vi "Get Current Log File Info.vi"(8 "error in (no error)":errorcluster, 10 "Session Name in":string, 11 "Data Logging Manager Ref in":T1) -> (0 "error out":errorcluster, 1 "Log File Path":path, 2 "Session Name out":string, 3 "Data Logging Manager Ref out":T1, 4 "Start Time":timestamp, 5 "Size":i64)   [LabVIEW 2020, in "NI_VS Data Logging API.lvlib"]
doc: "Gets information about the file to which <B>Session Name in</B> is currently logging data. If the session is not actively logging data to a file, <B>Log File Path</B> returns an empty array."
uses:
  <vilib>/NI VeriStand/Execution/DataLogging/NI_VS Data Logging API.lvlib
  <vilib>/NI VeriStand/Execution/DataLogging/IDataLogging Ref.ctl
  NationalInstruments.VeriStand.ClientAPI
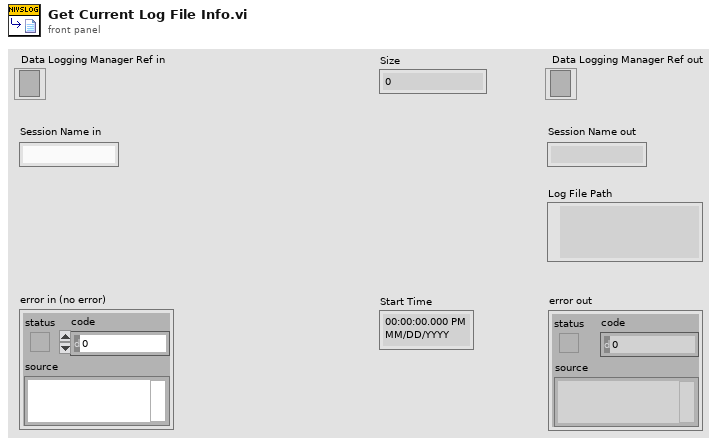
[diagram p1: front panel]
types:
  T1 = typedef "NI_VS Data Logging API.lvlib/IDataLogging Ref.ctl" = refnum<k24>
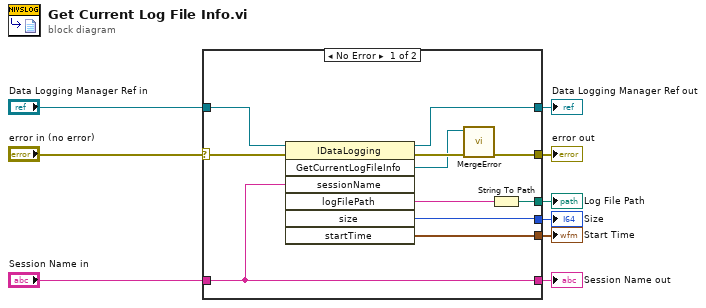
[diagram p0: block diagram]
diagram:
  n1 = case shown="No Error" "error in (no error)" {
    selector: "error in (no error)" -> [w18 w23]
    tunnel: [w15 w23] -> w8
    tunnel: [w14 w22] -> w7
    tunnel: "Data Logging Manager Ref in" -> [w20 w22]
    tunnel: [w19 w21] -> w5
    tunnel: "Session Name in" -> [w19 w21]
    tunnel: [w12 _] -> w3
    tunnel: [w11 _] -> w2
    tunnel: [w10 _] -> w1
    frame No Error {
      n2 = invoke class="IDataLogging" method="GetCurrentLogFileInfo"(reference=w20, error in=w18, "sessionName"=w19) -> (reference out=w14:T1, error out=w17:errorcluster, "GetCurrentLogFileInfo"=w16:refnum<k24>, "logFilePath"=w13:string, "size"=w11:i64, "startTime"=w10:timestamp)  [unwired: 4 in, 1 out]
      n3 = call <vilib>:"MergeError.vi"("error in (no error)"=w17, "Error"=w16) -> ("error out"=w15:errorcluster)  [unwired: 9 out]
      n4 = String To Path(string=w13) -> (path=w12:path)
    }
    frame Error {
    }
  }
  "Data Logging Manager Ref out" <- w7
  "error out" <- w8
  "Session Name out" <- w5
  "Log File Path" <- w3
  "Size" <- w2
  "Start Time" <- w1
